vi "Insert VIs by Pattern.vi"(4 "New Node Name":string="Errors", 6 "pattern":string, 7 "Application in":refnum<vi>, 8 "Tree Map in":T1, 9 "Root path":string, 10 "DQMH Lib In":refnum<vi>) -> (0 "Tree Map Out":T1)   [LabVIEW 2019, in "Panther Dashboard.lvlib"]
uses:
  Panther Dashboard.lvlib
  <vilib>/National Instruments/Tree Map/Tree Map Data.ctl
  Map Attribute--enum.ctl
  <vilib>/National Instruments/Tree Map/Tree Map.lvlib
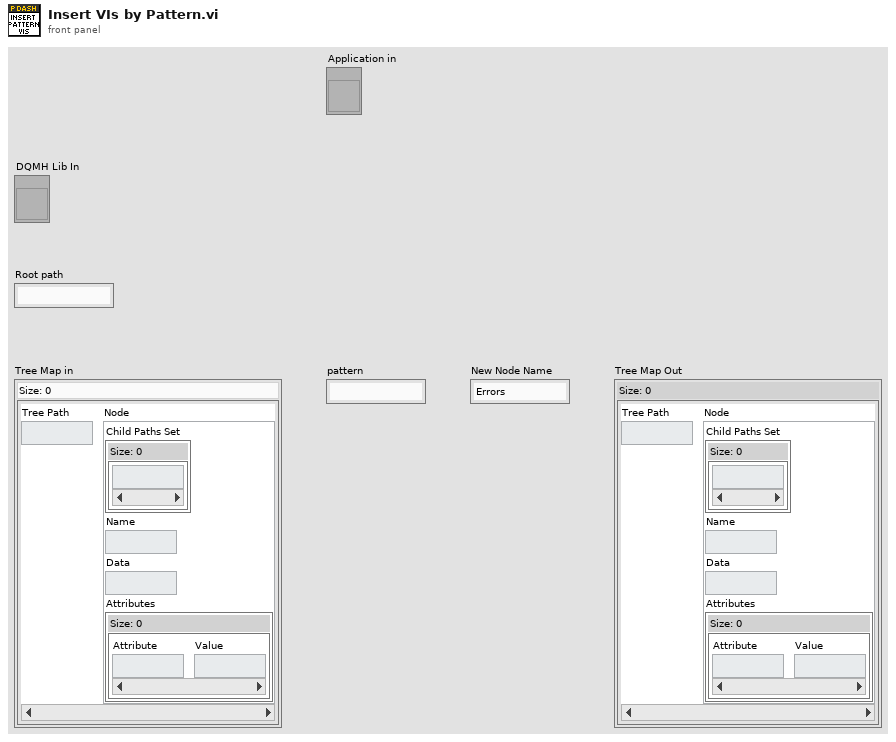
[diagram p1: front panel]
types:
  T1 = typedef "Tree Map.lvlib/Tree Map Data.ctl" = map{string, cluster{"Child Paths Set":set{string}, "Name":string, "Data":string, "Attributes":map{string, string}}}
  T2 = typedef "Panther Dashboard.lvlib/Map Attribute--enum.ctl" = enum16{"Path", "ModuleType", "Module Description", "Dependency?", "Target"}
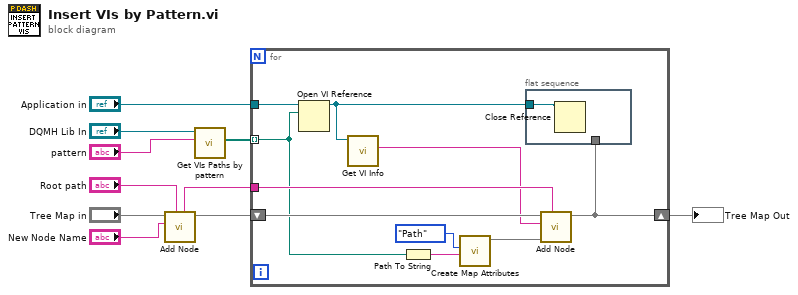
[diagram p0: block diagram]
diagram:
  n1 = call <vilib>:"Add Node.vi"("Parent Path"="Root path", "New Node Name"="New Node Name", "Tree Map In"="Tree Map in") -> ("Tree Map Out"=w6:T1, "New Node Path"=w4:string)  [unwired: 6 in, 1 out]
  n2 = call "Get VIs Paths by pattern.vi"("pattern"="pattern", "Library in"="DQMH Lib In") -> ("All Files in Dir"=w2:path[])  [unwired: 7 in, 2 out]
  n3 = for {
    tunnel: "Application in" -> [w20]
    shift-right: [w19] -> w9
    shift-left: w6 -> [w18]
    tunnel: w4 -> [w17]
    tunnel: w2 -> [w16] mode=indexing
    n4 = Open VI Reference(application reference (local)=w20, vi path=w16) -> (vi reference=w11:refnum<vi>)  [unwired: 4 in, 1 out]
    n5 = call "Get VI Info.vi"("VI in"=w11) -> ("Plain Name"=w15:string)  [unwired: 7 in, 3 out]
    n6 = Path To String(path=w16) -> (string=w13:string)
    n7 = call "Create Map Attributes.vi"("Attribute"=w13, "Map Attribute"=Map_Attribute--enum."Path") -> ("Root Attributes"=w12:map{string, string})  [unwired: 9 in]
    n8 = flat-sequence {
      tunnel: w11 -> [w21]
      tunnel: w19 -> [_]
      frame #0 {
        n9 = Close Reference(reference=w21) -> ()  [unwired: 1 in, 1 out]
      }
    }
    n10 = call <vilib>:"Add Node.vi"("Parent Path"=w17, "Attributes"=w12, "New Node Name"=w15, "Tree Map In"=w18) -> ("Tree Map Out"=w19:T1)  [unwired: 5 in, 2 out]
  }
  "Tree Map Out" <- w9
